vi "batchgenkey.vi"(0 "HGF_GPG in":refnum<class "HGF_GPG.lvclass">, 1 "options file":path, 2 "keyringfile":path, 3 "Sec keyringfile":path, 4 "password":string, 5 "error in (no error)":errorcluster, 6 "Name":string, 8 "Trust DB":path) -> (10 "dup Trust DB":path, 12 "Key-ID":string, 13 "success":bool, 14 "HGF_GPG out":refnum<class "HGF_GPG.lvclass">, 15 "dup options file":path, 16 "dup keyringfile":path, 17 "dup Sec keyringfile":path, 19 "error out":errorcluster)   [LabVIEW 2012, in "HGF_GPG.lvlib" / "HGF_GPG.lvclass"]
doc: "Generate a Key with a batch command. If no Password is set, the function uses a self-created. If no Name is set, the object's name will is used."
uses:
  HGF_GPG.lvclass
  HGF_GPG.lvclass/HGF_GPG.ctl
  HGF_BaseClasses/HGF_Factory/HGF_Factory.lvclass
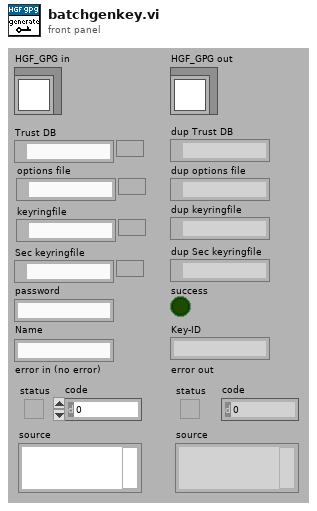
[diagram p1: front panel]
types:
  T1 = enum16{"open", "replace", "create", "open or create", "replace or create", "replace or create with confirmation"}
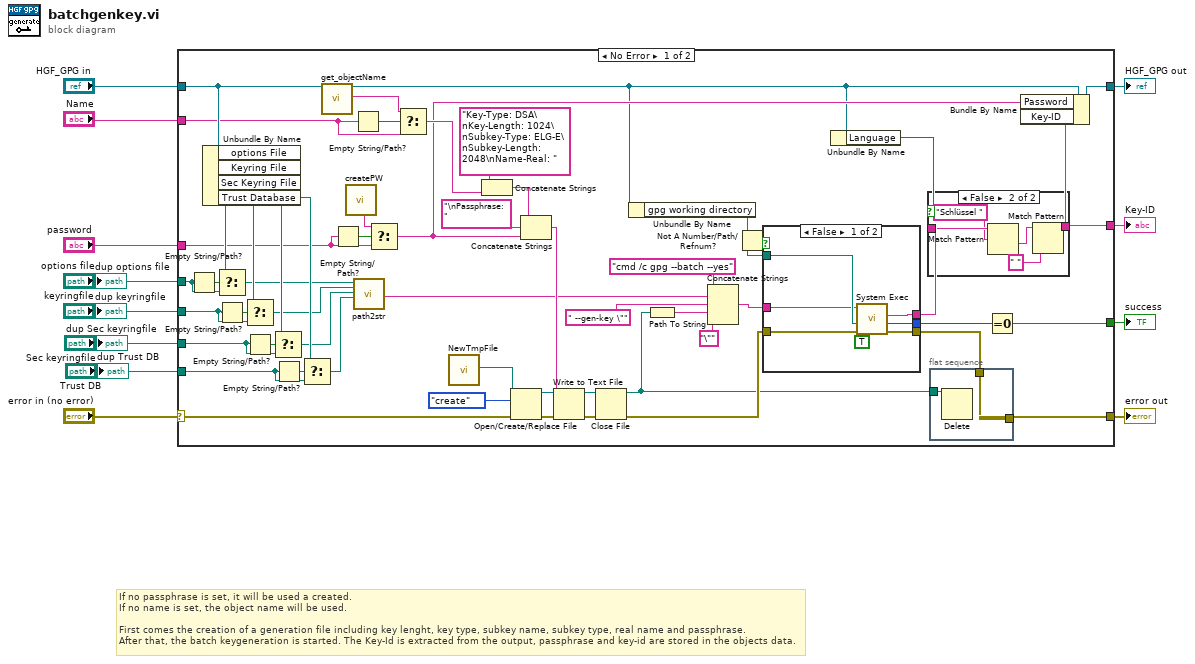
[diagram p0: block diagram]
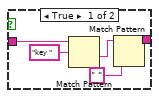
[diagram p2: hidden frame]
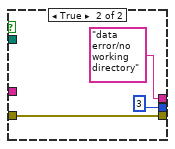
[diagram p3: hidden frame]
diagram:
  # "If no passphrase is set, it will be used a created.\nIf no name is set, the object name will be used.\n\nFirst comes the creation of a generation file including key lenght, key type, subkey name, subkey type, real name and passphrase.\nAfter that, the batch keygeneration is started. The Key-Id is extracted from the output, passphrase and key-id are stored in the objects data."
  n1 = case shown="No Error" "error in (no error)" {
    selector: "error in (no error)" -> [w53 w91]
    tunnel: [w43 w91] -> w11
    tunnel: [w38 w90] -> w9
    tunnel: "HGF_GPG in" -> [w67 w90]
    tunnel: "password" -> [w61 _]
    tunnel: "Name" -> [w35 _]
    tunnel: [w40 _] -> w6
    tunnel: [w33 _] -> w5
    tunnel: "keyringfile" -> [w22 _]
    tunnel: "options file" -> [w25 _]
    tunnel: "Sec keyringfile" -> [w19 _]
    tunnel: "Trust DB" -> [w16 _]
    frame No Error {
      n2 = Empty String/Path?(string/path=w25) -> (empty?=w26:bool)
      n3 = Unbundle By Name(w67) -> ("options File"=w64:path, "Keyring File"=w63:path, "Sec Keyring File"=w65:path, "Trust Database"=w66:path)
      n4 = Select(t=w64, s=w26, f=w25) -> (s? t:f=w23:path)
      n5 = Empty String/Path?(string/path=w22) -> (empty?=w24:bool)
      n6 = Select(t=w63, s=w24, f=w22) -> (s? t:f=w17:path)
      n7 = Empty String/Path?(string/path=w19) -> (empty?=w21:bool)
      n8 = Select(t=w65, s=w21, f=w19) -> (s? t:f=w20:path)
      n9 = Empty String/Path?(string/path=w16) -> (empty?=w18:bool)
      n10 = Select(t=w66, s=w18, f=w16) -> (s? t:f=w15:path)
      n11 = call "get_objectName.vi"("HGF_Factory"=w67) -> ("dup HGF_Factory"=w14:refnum<class "HGF_GPG.lvclass">, "objectName"=w36:string)  [unwired: 1 in, 16 out]
      n12 = Empty String/Path?(string/path=w61) -> (empty?=w62:bool)
      n13 = call "createPW.vi"() -> ("String"=w60:string)
      n14 = Empty String/Path?(string/path=w35) -> (empty?=w37:bool)
      n15 = call "path2str.vi"("options file"=w23, "keyringfile"=w17, "Sec keyringfile"=w20, "Trust DB"=w15) -> ("opt/keyr/seckeyr/trusdb"=w27:string)  [unwired: 2 in, 13 out]
      n16 = Select(t=w60, s=w62, f=w61) -> (s? t:f=w30:string)
      n17 = Select(t=w36, s=w37, f=w35) -> (s? t:f=w34:string)
      n18 = call "NewTmpFile.vi"() -> ("path"=w57:path)  [unwired: 1 in, 18 out]
      n19 = Concatenate Strings("Key-Type: DSA\nKey-Length: 1024\nSubkey-Type: ELG-E\nSubkey-Length: 2048\nName-Real: " ("string"), w34) -> (w32:string)
      n20 = Open/Create/Replace File(file path (use dialog)=w57, error in=w53, operation (0:open)=T1."create") -> (refnum out=w55:refnum<file>, error out=w54:errorcluster)  [unwired: 4 out]
      n21 = Concatenate Strings(w32, "\nPassphrase: " ("string"), w30) -> (w31:string)
      n22 = Write to Text File(file (use dialog)=w55, text=w31, error in=w54) -> (refnum out=w51:refnum<file>, error out=w52:errorcluster)  [unwired: 2 out]
      n23 = Close File(refnum=w51, error in=w52) -> (path=w42:path, error out=w44:errorcluster)
      n24 = Unbundle By Name(w14) -> ("gpg working directory"=w47:path)
      n25 = Path To String(path=w42) -> (string=w50:string)
      n26 = Concatenate Strings("cmd /c gpg --batch --yes", w27, " --gen-key \"" ("string"), w50, "\"") -> (w46:string)
      n27 = Not A Number/Path/Refnum?(number/path/refnum=w47) -> (NaN/Path/Refnum?=w48:bool)
      n28 = case shown="False" w48 {
        tunnel: w44 -> [w86 w89]
        tunnel: [w85 w89] -> w45
        tunnel: w47 -> [w84 _]
        tunnel: w46 -> [w81 _]
        tunnel: [w83 "data error/no working directory" ("standard error")] -> w39
        tunnel: [w82 3 ("return code")] -> w41
        frame False {
          n29 = call <vilib>:"System Exec.vi"("run minimized? (F)"=TRUE, "error in (no error)"=w86, "working directory"=w84, "command line"=w81) -> ("error out"=w85:errorcluster, "return code"=w82:i32, "standard error"=w83:string)  [unwired: 2 in, 3 out]
        }
        frame True {
        }
      }
      n30 = Unbundle By Name(w14) -> ("Language"=w13:bool)
      n31 = case shown="False" w13 {
        tunnel: w39 -> [w72 w77]
        tunnel: [w68 w73] -> w33
        frame True {
          n32 = Match Pattern(string=w72, regular expression="key ") -> (after substring=w70:string)  [unwired: 4 out]
          n33 = Match Pattern(string=w70, regular expression=" ") -> (before substring=w68:string)  [unwired: 4 out]
        }
        frame False {
          n34 = Match Pattern(string=w77, regular expression="Schlüssel ") -> (after substring=w75:string)  [unwired: 4 out]
          n35 = Match Pattern(string=w75, regular expression=" ") -> (before substring=w73:string)  [unwired: 4 out]
        }
      }
      n36 = flat-sequence {
        tunnel: w45 -> [w79]
        tunnel: [w79] -> w43
        tunnel: w42 -> [w78]
        frame #0 {
          n37 = Delete(path (use dialog)=w78) -> ()  [unwired: 1 in, 6 out]
        }
      }
      n38 = Equal To 0?(x=w41) -> (x = 0?=w40:bool)
      n39 = Bundle By Name(cluster=w14, "Password"=w30, "Key-ID"=w33) -> (w38:refnum<class "HGF_GPG.lvclass">)
    }
    frame Error {
    }
  }
  "error out" <- w11
  "HGF_GPG out" <- w9
  "success" <- w6
  "Key-ID" <- w5
  "dup options file" <- "options file"
  "dup keyringfile" <- "keyringfile"
  "dup Sec keyringfile" <- "Sec keyringfile"
  "dup Trust DB" <- "Trust DB"
